vi "predefined_entities2.vi"() -> ()   [LabVIEW 2021]
panel:
  in  "Resource Name":refnum<k15>="5842"
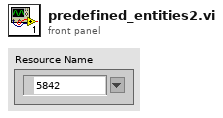
[diagram p1: front panel]
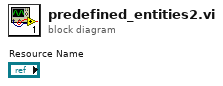
[diagram p0: block diagram]
diagram:
